vi "Write test.vi"(8 "error in (no error)":errorcluster, 10 "test":dbl, 11 "Test Channel in":refnum<class "Test Channel.lvclass">) -> (0 "error out":errorcluster, 3 "Test Channel out":refnum<class "Test Channel.lvclass">)   [LabVIEW 2021, in "Test Channel.lvclass"]
uses:
  Test Channel.lvclass
  Test Channel.lvclass/Test Channel.ctl
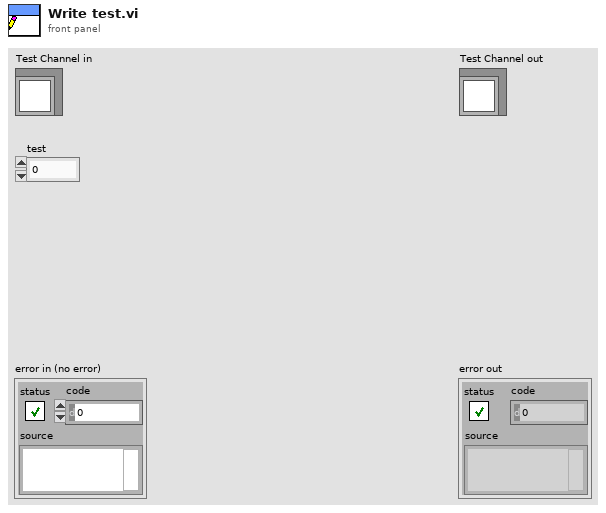
[diagram p1: front panel]
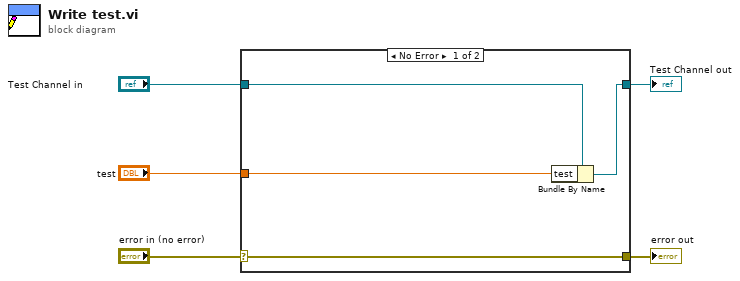
[diagram p0: block diagram]
diagram:
  n1 = case shown="No Error" "error in (no error)" {
    selector: "error in (no error)" -> [w9 w10]
    tunnel: [w9 w10] -> w4
    tunnel: [w7 w11] -> w2
    tunnel: "Test Channel in" -> [w8 w11]
    tunnel: "test" -> [w6 _]
    frame No Error {
      n2 = Bundle By Name(cluster=w8, "test"=w6) -> (w7:refnum<class "Test Channel.lvclass">)
    }
    frame Error {
    }
  }
  "error out" <- w4
  "Test Channel out" <- w2
